vi "SQLQueryWrapper.vi"() -> ()   [LabVIEW 2022 SP3]
uses:
  DataTypes/DBAction--Enum.ctl
  DataTypes/LocationStatus--Enum.ctl
  DataTypes/SlotPriority--Cluster.ctl
  DataTypes/SQLQuery--Enum.ctl
  DataTypes/Stocker--Enum.ctl
  DataTypes/Module--Cluster.ctl
  DataTypes/InventoryRecord--Cluster.ctl
panel:
  out "Data":string[][](array[string])
  in  "Table":string
  in  "InventoryRecord":T1 {"Stocker" items=["Main", "Exp1", "Exp2"]}
  in  "Query":T5
  out "Error out":errorcluster
  in  "Error in (no error)":errorcluster
  out "Connection Out":refnum<k7>
  in  "Connection In":refnum<k7>
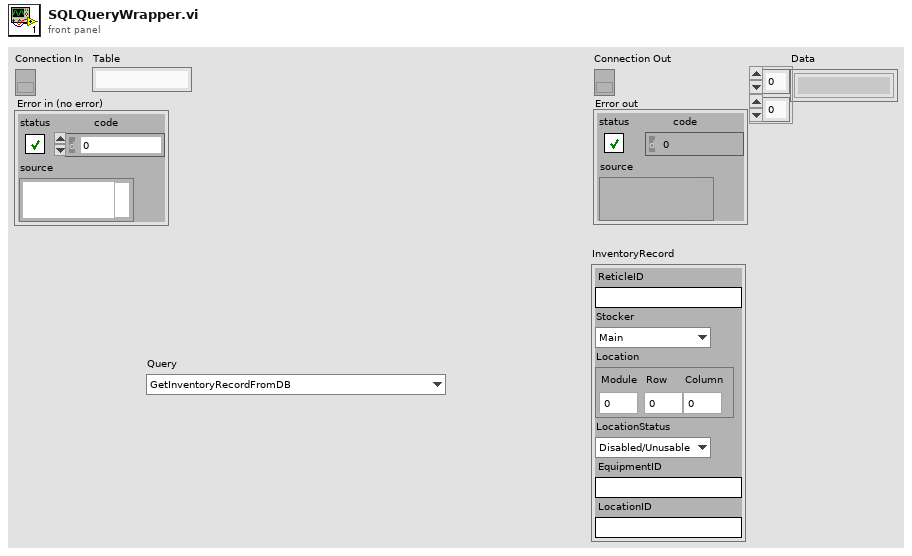
[diagram p1: front panel]
types:
  T1 = typedef "InventoryRecord--Cluster.ctl" = cluster{"ReticleID":string, "Stocker":T2, "Location":T3, "LocationStatus":T4, "EquipmentID":string, "LocationID":string}
  T2 = typedef "Stocker--Enum.ctl" = u16
  T3 = typedef "Module--Cluster.ctl" = cluster{"Module":u16, "Row":u16, "Column":u16}
  T4 = typedef "LocationStatus--Enum.ctl" = enum16{"Disabled/Unusable", "Full", "Empty"}
  T5 = typedef "SQLQuery--Enum.ctl" = enum16{"GetInventoryRecordFromDB", "GetReticleInfoFromDB", "GetLocationStatusFromDB", "UpdateInventoryRecord", "UpdateLocationStatus", "UpdateReticleLocationStatus", "AddReticleInDB", "RemoveReticleAtLocation", "RemoveReticleUsingReticleID", "GetLocationForReticleID", "GetAllLocations", "GetAllEmptyLocations", "GetAllLocationsInStocker", "GetAllFullLocations", "GetAllFullLocationsInStocker", "GetAllDisabledLocations", "GetAllDisabledLocationsInStocker", "FindFirstSlot"}
  T6 = typedef "SlotPriority--Cluster.ctl" = cluster{"Stocker":string, "Modules":i32[]}
  T7 = typedef "DBAction--Enum.ctl" = enum16{"Select", "Update"}
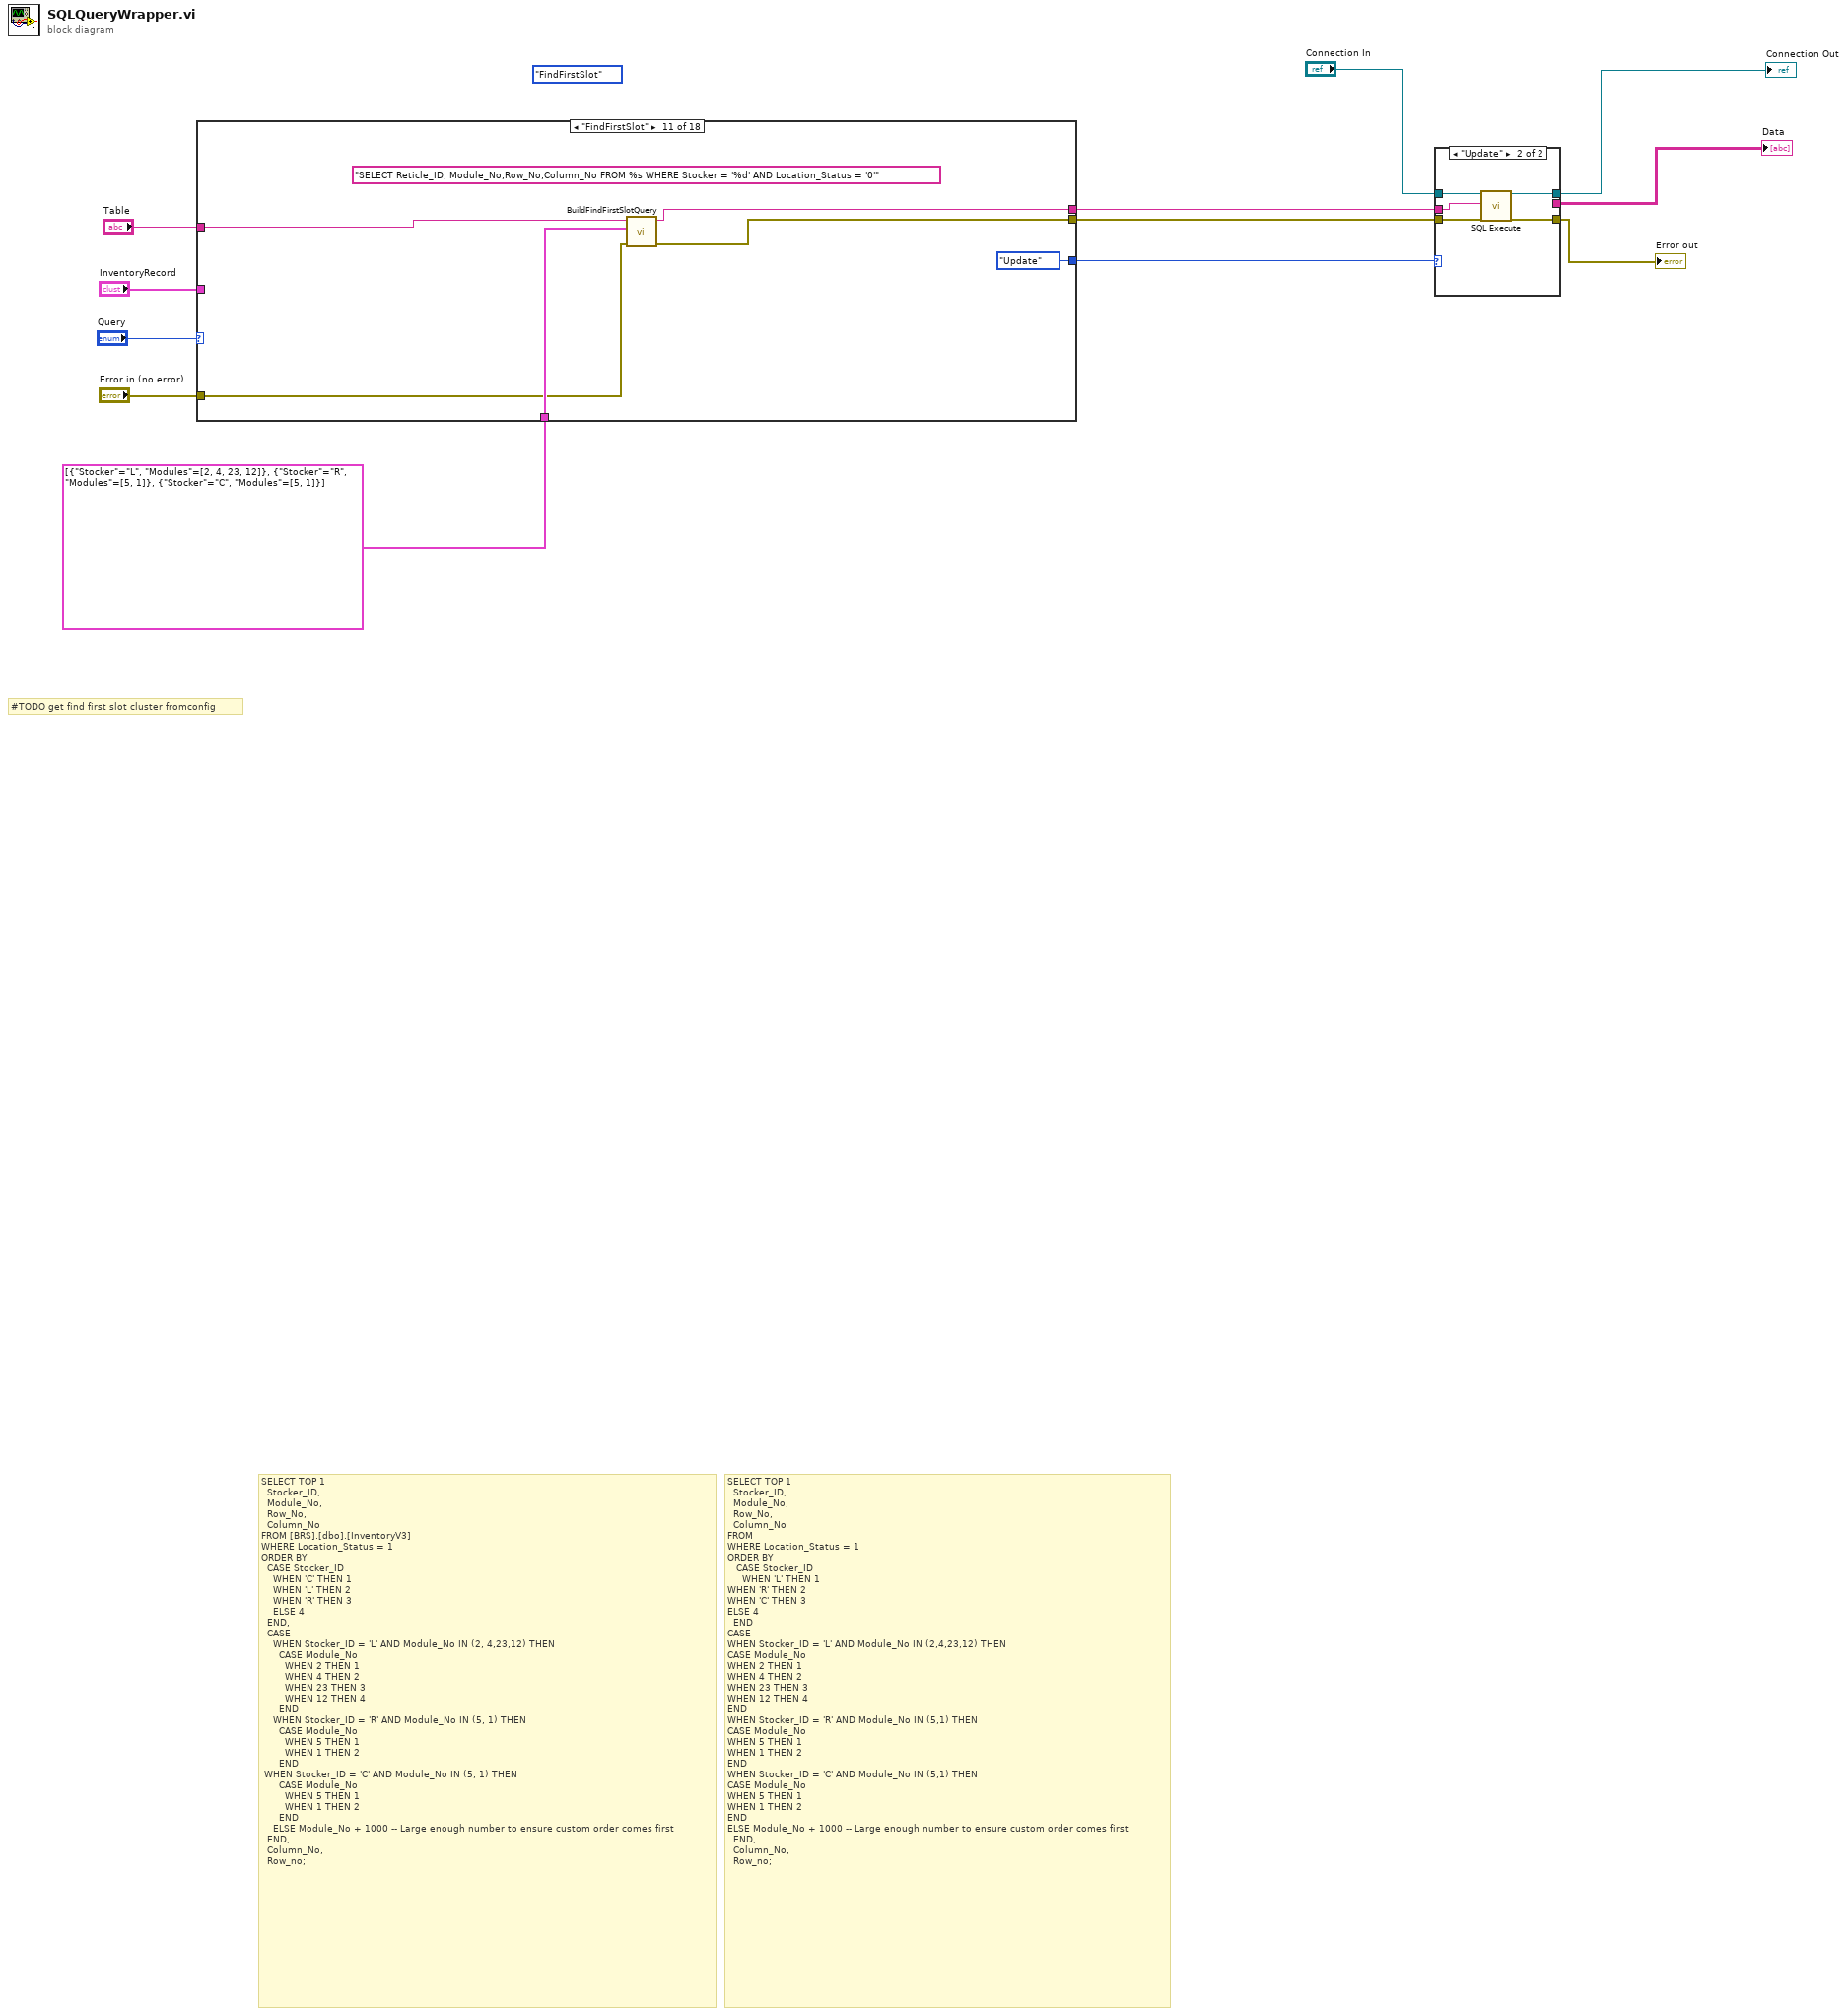
[diagram p0: block diagram]
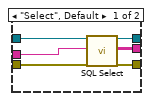
[diagram p2: hidden frame]
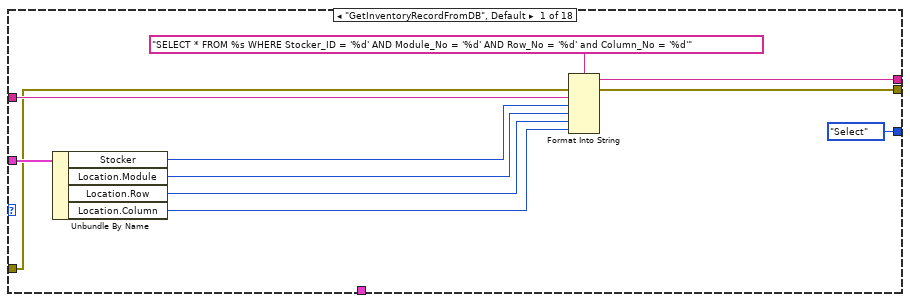
[diagram p3: hidden frame]
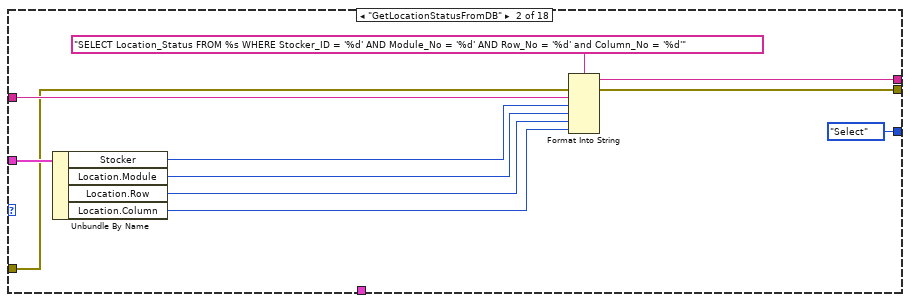
[diagram p4: hidden frame]
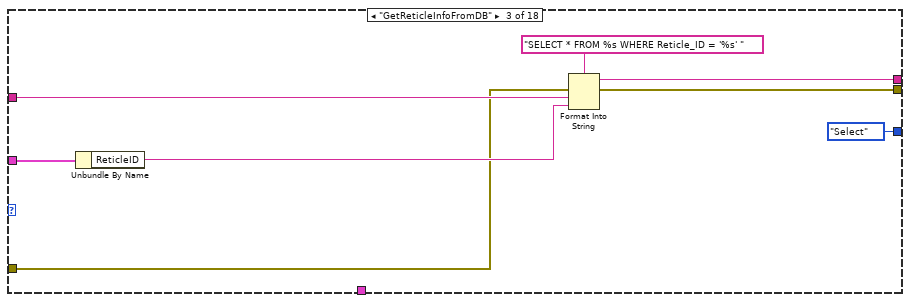
[diagram p5: hidden frame]
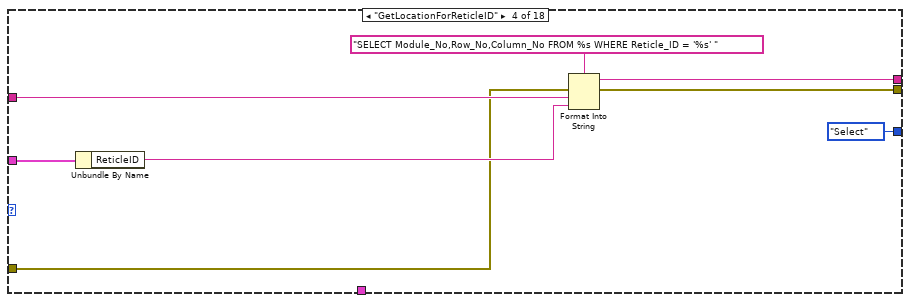
[diagram p6: hidden frame]
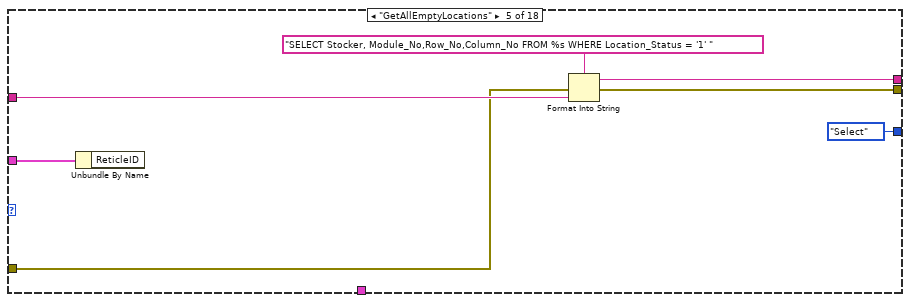
[diagram p7: hidden frame]
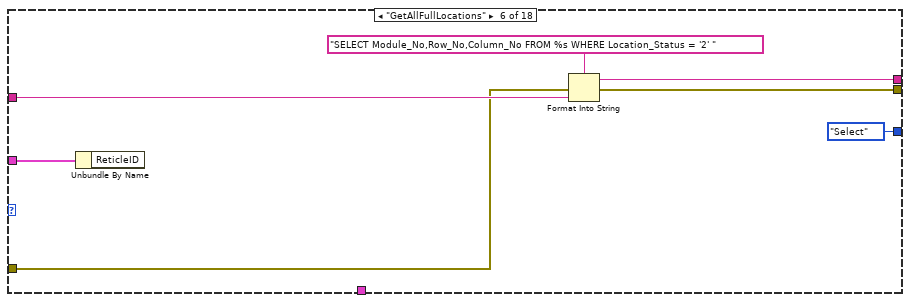
[diagram p8: hidden frame]
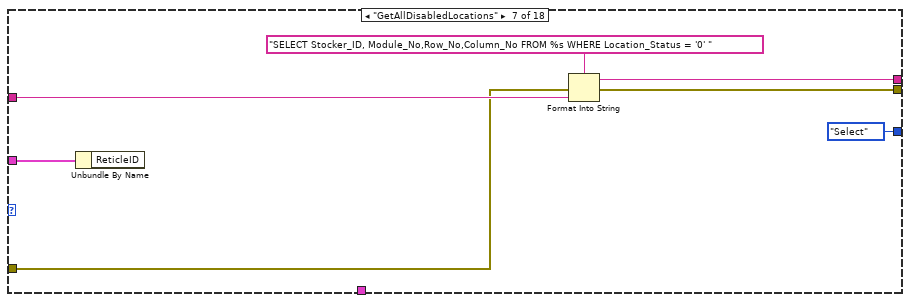
[diagram p9: hidden frame]
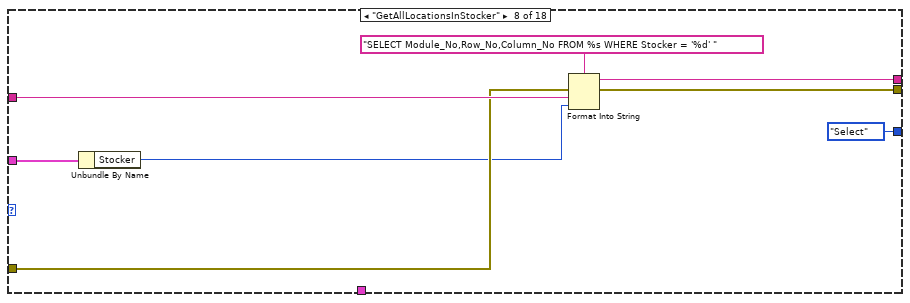
[diagram p10: hidden frame]
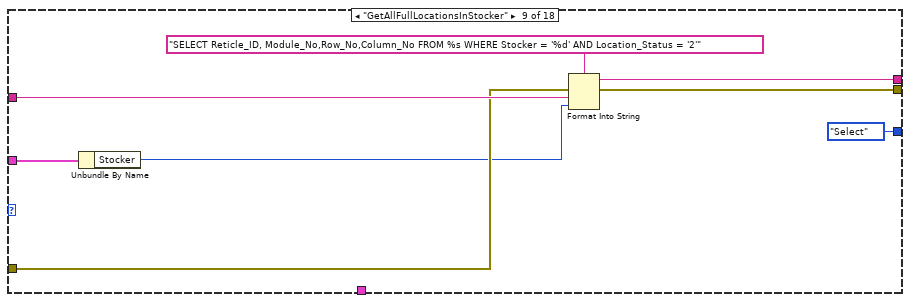
[diagram p11: hidden frame]
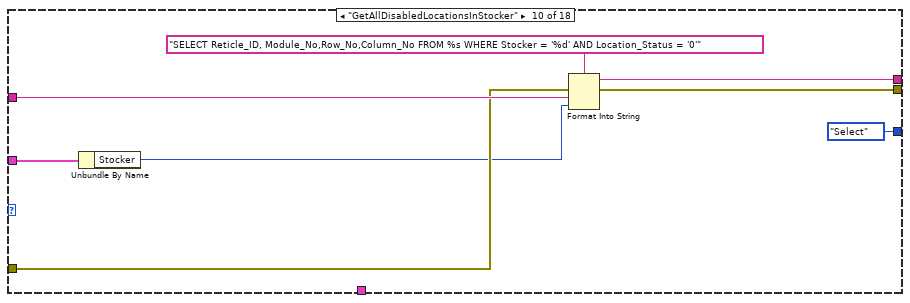
[diagram p12: hidden frame]
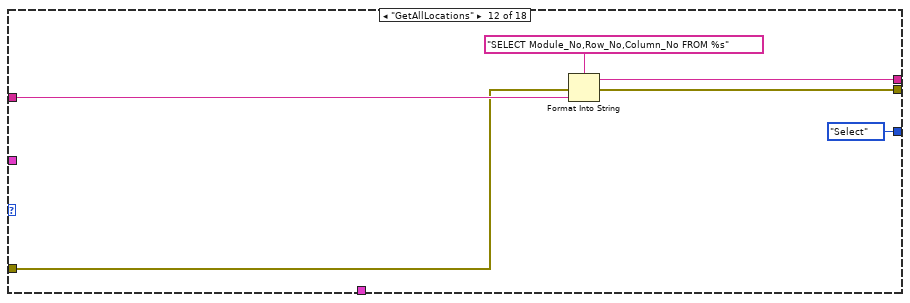
[diagram p13: hidden frame]
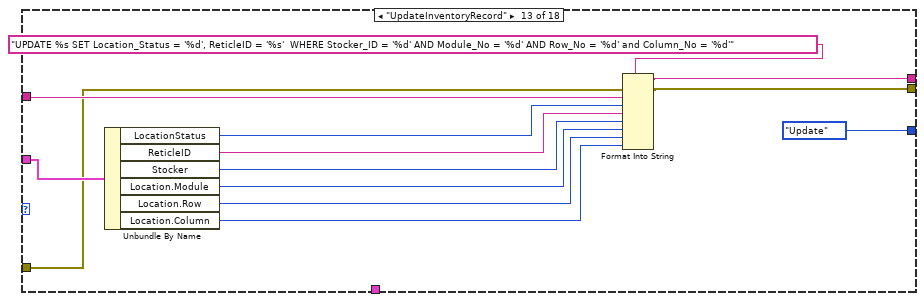
[diagram p14: hidden frame]
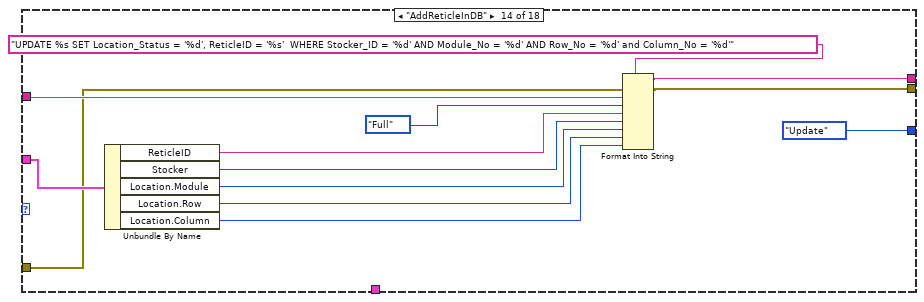
[diagram p15: hidden frame]
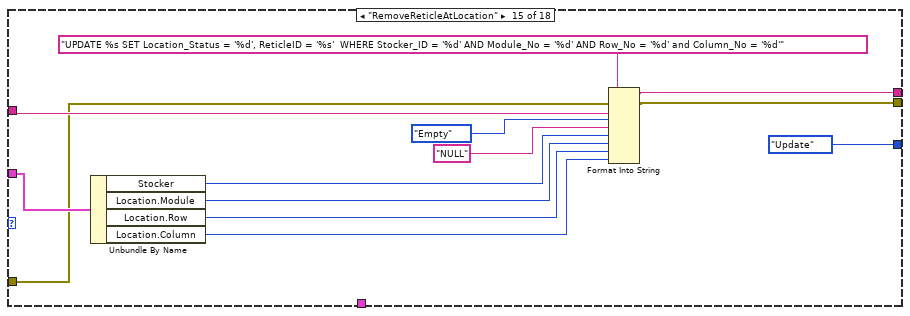
[diagram p16: hidden frame]
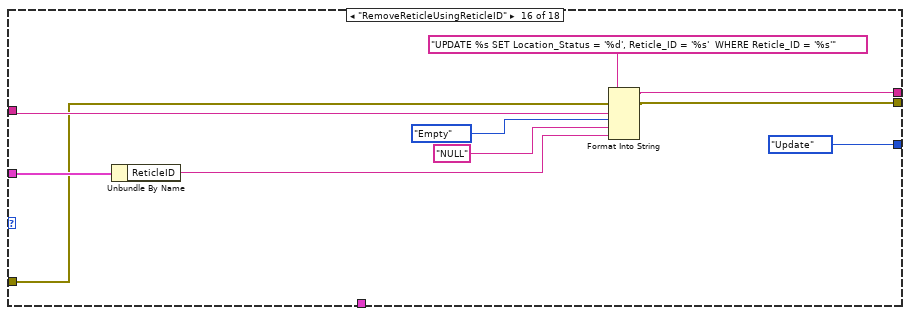
[diagram p17: hidden frame]
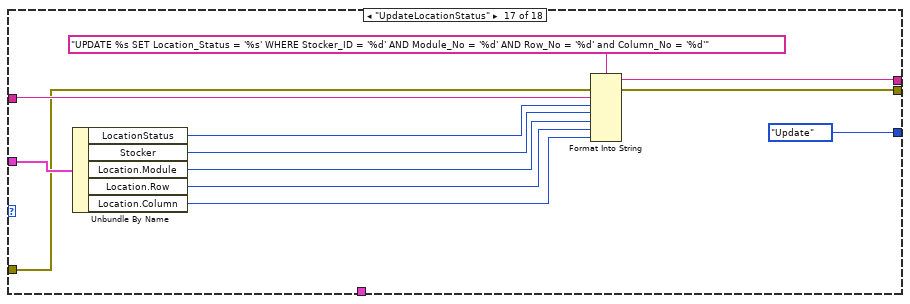
[diagram p18: hidden frame]
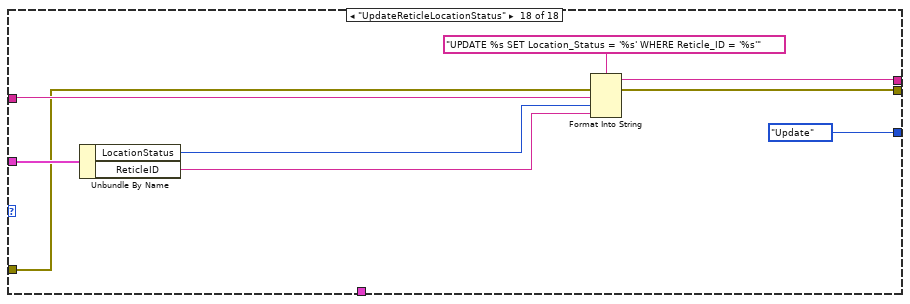
[diagram p19: hidden frame]
diagram:
  (unwired) SQLQuery--Enum."FindFirstSlot" ("Query")
  # "#TODO get find first slot cluster fromconfig"
  # "SELECT TOP 1 \n  Stocker_ID,\n  Module_No,\n  Row_No,\n  Column_No\nFROM \nWHERE Location_Status = 1\nORDER BY\n   CASE Stocker_ID\n     WHEN 'L' THEN 1\nWHEN 'R' THEN 2\nWHEN 'C' THEN 3\nELSE 4\n  END\nCASE\nWHEN Stocker_ID = 'L' AND Module_No IN (2,4,23,12) THEN\nCASE Module_No\nWHEN 2 THEN 1\nWHEN 4 THEN 2\nWHEN 23 THEN 3\nWHEN 12 THEN 4\nEND\nWHEN Stocker_ID = 'R' AND Module_No IN (5,1) THEN\nCASE Module_No\nWHEN 5 THEN 1\nWHEN 1 THEN 2\nEND\nWHEN Stocker_ID = 'C' AND Module_No IN (5,1) THEN\nCASE Module_No\nWHEN 5 THEN 1\nWHEN 1 THEN 2\nEND\nELSE Module_No + 1000 -- Large enough number to ensure custom order comes first\n  END,\n  Column_No,\n  Row_no;"
  # "SELECT TOP 1 \n  Stocker_ID,\n  Module_No,\n  Row_No,\n  Column_No\nFROM [BRS].[dbo].[InventoryV3]\nWHERE Location_Status = 1\nORDER BY\n  CASE Stocker_ID\n    WHEN 'C' THEN 1\n    WHEN 'L' THEN 2\n    WHEN 'R' THEN 3\n    ELSE 4\n  END,\n  CASE\n    WHEN Stocker_ID = 'L' AND Module_No IN (2, 4,23,12) THEN\n      CASE Module_No\n        WHEN 2 THEN 1\n        WHEN 4 THEN 2\n\t\t      WHEN 23 THEN 3\n\t       WHEN 12 THEN 4\n      END\n    WHEN Stocker_ID = 'R' AND Module_No IN (5, 1) THEN\n      CASE Module_No\n        WHEN 5 THEN 1\n        WHEN 1 THEN 2\n      END\n\tWHEN Stocker_ID = 'C' AND Module_No IN (5, 1) THEN\n      CASE Module_No\n        WHEN 5 THEN 1\n        WHEN 1 THEN 2\n      END\n    ELSE Module_No + 1000 -- Large enough number to ensure custom order comes first\n  END,\n  Column_No,\n  Row_no;"
  n1 = case shown="\"FindFirstSlot\"" "Query" {
    tunnel: "InventoryRecord" -> [w23 w34 w42 w50 w57 w64 w71 w79 w87 w95 _ _ w114 w128 w141 w154 w162 w173]
    tunnel: "Table" -> [w21 w32 w40 w48 w55 w62 w69 w77 w85 w93 w99 w106 w113 w127 w140 w153 w163 w174]
    tunnel: [w16 w27 w38 w46 w54 w61 w68 w76 w84 w92 w98 w105 w110 w124 w137 w150 w159 w170] -> w8
    tunnel: [w15 w26 w37 w45 w53 w60 w67 w75 w83 w91 w97 w104 w111 w125 w138 w151 w160 w171] -> w7
    tunnel: "Error in (no error)" -> [w14 w25 w36 w44 w52 w59 w66 w74 w82 w90 w96 w103 w112 w126 w139 w152 w161 w172]
    tunnel: [DBAction--Enum."Select" ("DBAction") DBAction--Enum."Select" ("DBAction") DBAction--Enum."Select" ("DBAction") DBAction--Enum."Select" ("DBAction") DBAction--Enum."Select" ("DBAction") DBAction--Enum."Select" ("DBAction") DBAction--Enum."Select" ("DBAction") DBAction--Enum."Select" ("DBAction") DBAction--Enum."Select" ("DBAction") DBAction--Enum."Select" ("DBAction") DBAction--Enum."Update" ("DBAction") DBAction--Enum."Select" ("DBAction") DBAction--Enum."Update" ("DBAction") DBAction--Enum."Update" ("DBAction") DBAction--Enum."Update" ("DBAction") DBAction--Enum."Update" ("DBAction") DBAction--Enum."Update" ("DBAction") DBAction--Enum."Update" ("DBAction")] -> w4
    tunnel: T6[] [{"Stocker"="L", "Modules"=[2, 4, 23, 12]}, {"Stocker"="R", "Modules"=[5, 1]}, {"Stocker"="C", "Modules"=[5, 1]}] -> [_ _ _ _ _ _ _ _ _ _ w100 _ _ _ _ _ _ _]
    frame "GetInventoryRecordFromDB", Default {
      n2 = Unbundle By Name(w23) -> ("Stocker"=w20:T2, "Location.Module"=w19:u16, "Location.Row"=w18:u16, "Location.Column"=w17:u16)
      n3 = Format Into String(format string="SELECT * FROM %s WHERE Stocker_ID = '%d' AND Module_No = '%d' AND Row_No = '%d' and Column_No = '%d'", error in=w14, w21, w20, w19, w18, w17) -> (resulting string=w16:string, error out=w15:errorcluster)  [unwired: 1 in]
    }
    frame "GetLocationStatusFromDB" {
      n4 = Unbundle By Name(w34) -> ("Stocker"=w31:T2, "Location.Module"=w30:u16, "Location.Row"=w29:u16, "Location.Column"=w28:u16)
      n5 = Format Into String(format string="SELECT Location_Status FROM %s WHERE Stocker_ID = '%d' AND Module_No = '%d' AND Row_No = '%d' and Column_No = '%d'", error in=w25, w32, w31, w30, w29, w28) -> (resulting string=w27:string, error out=w26:errorcluster)  [unwired: 1 in]
    }
    frame "GetReticleInfoFromDB" {
      n6 = Unbundle By Name(w42) -> ("ReticleID"=w39:string)
      n7 = Format Into String(format string="SELECT * FROM %s WHERE Reticle_ID = '%s' ", error in=w36, w40, w39) -> (resulting string=w38:string, error out=w37:errorcluster)  [unwired: 1 in]
    }
    frame "GetLocationForReticleID" {
      n8 = Unbundle By Name(w50) -> ("ReticleID"=w47:string)
      n9 = Format Into String(format string="SELECT Module_No,Row_No,Column_No FROM %s WHERE Reticle_ID = '%s' ", error in=w44, w48, w47) -> (resulting string=w46:string, error out=w45:errorcluster)  [unwired: 1 in]
    }
    frame "GetAllEmptyLocations" {
      n10 = Unbundle By Name(w57) -> ()  [unwired: 1 out]
      n11 = Format Into String(format string="SELECT Stocker, Module_No,Row_No,Column_No FROM %s WHERE Location_Status = '1' ", error in=w52, w55) -> (resulting string=w54:string, error out=w53:errorcluster)  [unwired: 1 in]
    }
    frame "GetAllFullLocations" {
      n12 = Unbundle By Name(w64) -> ()  [unwired: 1 out]
      n13 = Format Into String(format string="SELECT Module_No,Row_No,Column_No FROM %s WHERE Location_Status = '2' ", error in=w59, w62) -> (resulting string=w61:string, error out=w60:errorcluster)  [unwired: 1 in]
    }
    frame "GetAllDisabledLocations" {
      n14 = Unbundle By Name(w71) -> ()  [unwired: 1 out]
      n15 = Format Into String(format string="SELECT Stocker_ID, Module_No,Row_No,Column_No FROM %s WHERE Location_Status = '0' ", error in=w66, w69) -> (resulting string=w68:string, error out=w67:errorcluster)  [unwired: 1 in]
    }
    frame "GetAllLocationsInStocker" {
      n16 = Unbundle By Name(w79) -> ("Stocker"=w72:T2)
      n17 = Format Into String(format string="SELECT Module_No,Row_No,Column_No FROM %s WHERE Stocker = '%d' ", error in=w74, w77, w72) -> (resulting string=w76:string, error out=w75:errorcluster)  [unwired: 1 in]
    }
    frame "GetAllFullLocationsInStocker" {
      n18 = Unbundle By Name(w87) -> ("Stocker"=w80:T2)
      n19 = Format Into String(format string="SELECT Reticle_ID, Module_No,Row_No,Column_No FROM %s WHERE Stocker = '%d' AND Location_Status = '2'", error in=w82, w85, w80) -> (resulting string=w84:string, error out=w83:errorcluster)  [unwired: 1 in]
    }
    frame "GetAllDisabledLocationsInStocker" {
      n20 = Unbundle By Name(w95) -> ("Stocker"=w88:T2)
      n21 = Format Into String(format string="SELECT Reticle_ID, Module_No,Row_No,Column_No FROM %s WHERE Stocker = '%d' AND Location_Status = '0'", error in=w90, w93, w88) -> (resulting string=w92:string, error out=w91:errorcluster)  [unwired: 1 in]
    }
    frame "FindFirstSlot" {
      (unwired) "SELECT Reticle_ID, Module_No,Row_No,Column_No FROM %s WHERE Stocker = '%d' AND Location_Status = '0'" ("format string")
      n22 = call "BuildFindFirstSlotQuery.vi"("error in (no error)"=w96, "Array"=w100, "Table"=w99) -> ("error out"=w97:errorcluster, "String"=w98:string)  [unwired: 7 in]
    }
    frame "GetAllLocations" {
      n23 = Format Into String(format string="SELECT Module_No,Row_No,Column_No FROM %s", error in=w103, w106) -> (resulting string=w105:string, error out=w104:errorcluster)  [unwired: 1 in]
    }
    frame "UpdateInventoryRecord" {
      n24 = Unbundle By Name(w114) -> ("LocationStatus"=w116:T4, "ReticleID"=w108:string, "Stocker"=w115:T2, "Location.Module"=w119:u16, "Location.Row"=w118:u16, "Location.Column"=w117:u16)
      n25 = Format Into String(format string="UPDATE %s SET Location_Status = '%d', ReticleID = '%s'  WHERE Stocker_ID = '%d' AND Module_No = '%d' AND Row_No = '%d' and Column_No = '%d'", error in=w112, w113, w116, w108, w115, w119, w118, w117) -> (resulting string=w110:string, error out=w111:errorcluster)  [unwired: 1 in]
    }
    frame "AddReticleInDB" {
      n26 = Unbundle By Name(w128) -> ("ReticleID"=w122:string, "Stocker"=w129:T2, "Location.Module"=w132:u16, "Location.Row"=w131:u16, "Location.Column"=w130:u16)
      n27 = Format Into String(format string="UPDATE %s SET Location_Status = '%d', ReticleID = '%s'  WHERE Stocker_ID = '%d' AND Module_No = '%d' AND Row_No = '%d' and Column_No = '%d'", error in=w126, w127, LocationStatus--Enum."Full" ("LocationStatus"), w122, w129, w132, w131, w130) -> (resulting string=w124:string, error out=w125:errorcluster)  [unwired: 1 in]
    }
    frame "RemoveReticleAtLocation" {
      n28 = Unbundle By Name(w141) -> ("Stocker"=w142:T2, "Location.Module"=w145:u16, "Location.Row"=w144:u16, "Location.Column"=w143:u16)
      n29 = Format Into String(format string="UPDATE %s SET Location_Status = '%d', ReticleID = '%s'  WHERE Stocker_ID = '%d' AND Module_No = '%d' AND Row_No = '%d' and Column_No = '%d'", error in=w139, w140, LocationStatus--Enum."Empty" ("LocationStatus"), "NULL" ("input 3"), w142, w145, w144, w143) -> (resulting string=w137:string, error out=w138:errorcluster)  [unwired: 1 in]
    }
    frame "RemoveReticleUsingReticleID" {
      n30 = Unbundle By Name(w154) -> ("ReticleID"=w155:string)
      n31 = Format Into String(format string="UPDATE %s SET Location_Status = '%d', Reticle_ID = '%s'  WHERE Reticle_ID = '%s'", error in=w152, w153, LocationStatus--Enum."Empty" ("LocationStatus"), "NULL" ("input 3"), w155) -> (resulting string=w150:string, error out=w151:errorcluster)  [unwired: 1 in]
    }
    frame "UpdateLocationStatus" {
      n32 = Unbundle By Name(w162) -> ("LocationStatus"=w158:T4, "Stocker"=w157:T2, "Location.Module"=w166:u16, "Location.Row"=w165:u16, "Location.Column"=w164:u16)
      n33 = Format Into String(format string="UPDATE %s SET Location_Status = '%s' WHERE Stocker_ID = '%d' AND Module_No = '%d' AND Row_No = '%d' and Column_No = '%d'", error in=w161, w163, w158, w157, w166, w165, w164) -> (resulting string=w159:string, error out=w160:errorcluster)  [unwired: 1 in]
    }
    frame "UpdateReticleLocationStatus" {
      n34 = Unbundle By Name(w173) -> ("LocationStatus"=w169:T4, "ReticleID"=w175:string)
      n35 = Format Into String(format string="UPDATE %s SET Location_Status = '%s' WHERE Reticle_ID = '%s'", error in=w172, w174, w169, w175) -> (resulting string=w170:string, error out=w171:errorcluster)  [unwired: 1 in]
    }
  }
  n36 = case shown="\"Update\"" w4 {
    tunnel: "Connection In" -> [w183 w188]
    tunnel: [w182 w184] -> w11
    tunnel: [w181 w185] -> w10
    tunnel: w8 -> [w180 w187]
    tunnel: w7 -> [w179 w186]
    tunnel: [w178 _] -> w5
    frame "Select", Default {
      n37 = call "SQL Select.vi"("Connection In"=w183, "SQL Query"=w180, "Error in (no error)"=w179) -> ("Connection Out"=w182:refnum<k7>, "Data"=w178:string[][], "Error out"=w181:errorcluster)  [unwired: 14 in]
    }
    frame "Update" {
      n38 = call "SQL Execute.vi"("Connection In"=w188, "SQL Query"=w187, "Error in (no error)"=w186) -> ("Connection Out"=w184:refnum<k7>, "Error out"=w185:errorcluster)  [unwired: 15 in]
    }
  }
  "Connection Out" <- w11
  "Error out" <- w10
  "Data" <- w5
